vi "subSetParameters(HL).vi"(0 "IVI Refnum in":refnum<k15>, 5 "Rx Parameters":T1, 11 "error in (no error)":errorcluster) -> (4 "IVI Refnum out":refnum<k15>, 6 "samples per acquisition":i32, 8 "Frame Parameters":T2 {"Acq Duration [sec]" min=0.0 step=0.001 format="%#.6p"; "Stop Carrier [Hz]" min=50000000.0 max=6000000000.0 step=1000.0 format="%#.15p"; "Start Carrier [Hz]" min=50000000.0 max=6000000000.0 step=1000.0 format="%#.15p"}, 10 "test carrier frequencies":dbl[](array[numeric]), 15 "error out":errorcluster)   [LabVIEW 2011]
uses:
  subFrameParams.ctl
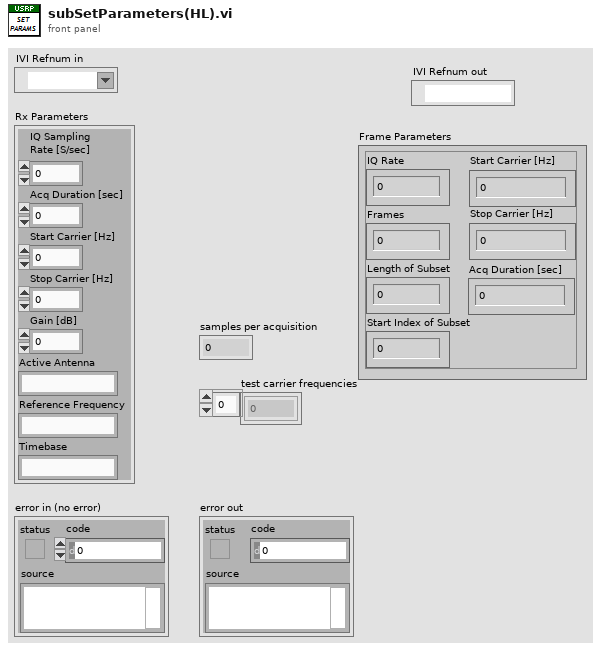
[diagram p1: front panel]
types:
  T1 = cluster{"IQ Sampling\nRate [S/sec]":dbl, "Acq Duration [sec]":dbl, "Start Carrier [Hz]":dbl, "Stop Carrier [Hz]":dbl, "Gain [dB]":dbl, "Active Antenna":string, "Reference Frequency":string, "Timebase":string}
  T2 = typedef "subFrameParams.ctl" = cluster{"IQ Rate":dbl, "Frames":i32, "Length of Subset":i32, "Start Index of Subset":i32, "Start Carrier [Hz]":dbl, "Stop Carrier [Hz]":dbl, "Acq Duration [sec]":dbl}
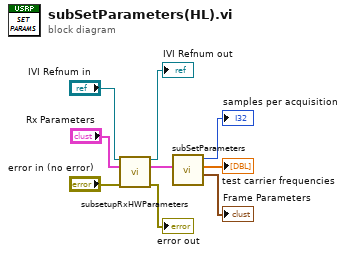
[diagram p0: block diagram]
diagram:
  n1 = call "subsetupRxHWParameters.vi"("IVI Refnum in"="IVI Refnum in", "Rx Parameters"="Rx Parameters", "error in (no error)"="error in (no error)") -> ("IVI Refnum out"=→"IVI Refnum out":refnum<k15>, "Rx Parameters"=w7:T1, "error out"=→"error out":errorcluster)  [unwired: 10 in]
  n2 = call "subSetParameters.vi"("Rx Parameters"=w7) -> ("Frame Parameters"=→"Frame Parameters":T2, "test carrier frequencies"=→"test carrier frequencies":dbl[], "samples per acquisition"=→"samples per acquisition":i32)  [unwired: 8 in]
